vi "IMAQController.ReadConfigFile.vi"(0 "object ref in":refnum<vi>, 5 "error in":errorcluster) -> (14 "object ref out":refnum<vi>, 16 "Camera-System Configuration":T1(array[cluster]), 19 "error out":errorcluster)   [LabVIEW 2014, in "IMAQController.lvlib"]
uses:
  IMAQController.lvlib
  CSCore/BaseProcess/BaseProcess.lvlib
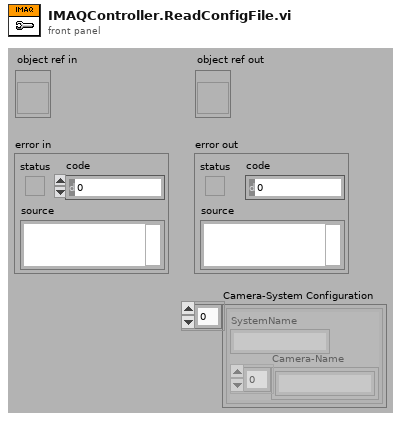
[diagram p1: front panel]
types:
  T1 = cluster{"SystemName":string, "Camera-Name":string[]}[]
  T2 = cluster{"SystemName":string, "Camera-Name":string[]}
  T3 = typedef "BaseProcess.lvlib/BaseProcess.i attribute.ctl" = cluster{"EventStatus":string, "EventError":i32, "PresetEvtWatchD":i32, "PresetPdcWatchD":i32, "EventTimeout":i32, "PeriodicInterval":i32, "Interface":string[], "Address":string[], "Special":string[], "PeriodicError":i32, "PeriodicStatus":string, "SuperProc":string, "Descriptors":T4[], "CaseRef":refnum<vi>, "PdcRef":refnum<vi>, "Thread Ref":refnum<vi>, "eventErrorID":i32, "eventStatusID":i32, "periodicErrorID":i32, "periodicStatusID":i32, "pdcCtrID":i32}
  T4 = typedef "BaseProcess.lvlib/BaseProcess.descriptor definition.ctl" = cluster{"selector":string, "descriptor":T5}
  T5 = typedef "BaseProcess.lvlib/BaseProcess.descriptor string definition.ctl" = string
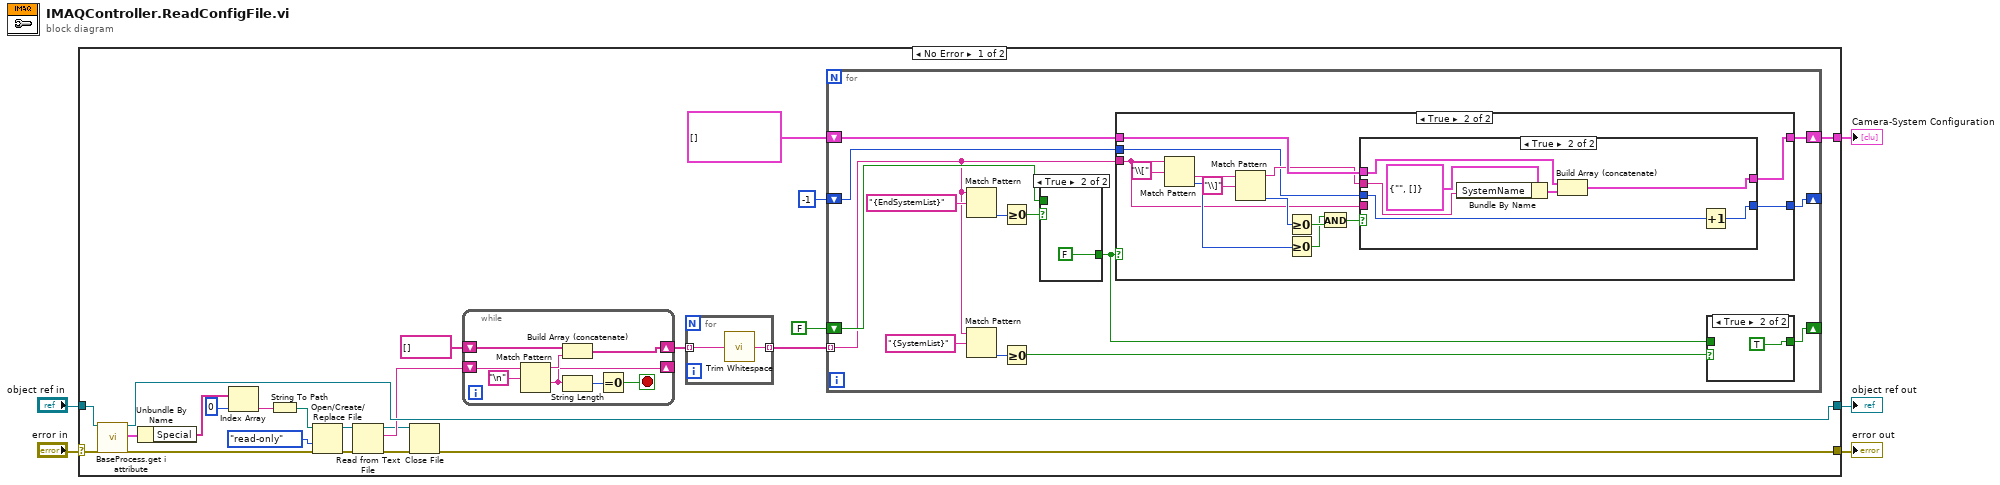
[diagram p0: block diagram]
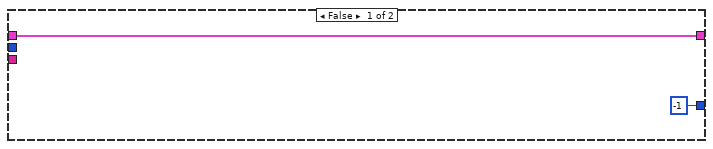
[diagram p2: hidden frame]
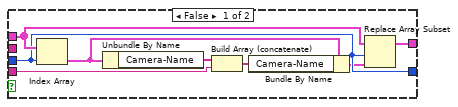
[diagram p3: hidden frame]
diagram:
  n1 = case shown="No Error" "error in" {
    selector: "error in" -> [w27 w89]
    tunnel: "object ref in" -> [w28 w88]
    tunnel: [w11 w89] -> w3
    tunnel: [w22 w88] -> w2
    tunnel: [w6 _] -> w1
    frame No Error {
      n2 = call "BaseProcess.get i attribute.vi"("i ref in"=w28, "error in (no error)"=w27) -> ("i ref out"=w22:refnum<vi>, "i attribute"=w26:T3, "error out"=w21:errorcluster)  [unwired: 15 in]
      n3 = Unbundle By Name(w26) -> ("Special"=w25:string[])
      n4 = Index Array(array=w25, index=0) -> (element=w23:string)
      n5 = String To Path(string=w23) -> (path=w20:path)
      n6 = Open/Create/Replace File(file path (use dialog)=w20, error in=w21, access (0:read/write)=enum16{"read/write", "read-only", "write-only"}."read-only") -> (refnum out=w17:refnum<file>, error out=w18:errorcluster)  [unwired: 3 in, 1 out]
      n7 = Read from Text File(file (use dialog)=w17, error in=w18) -> (refnum out=w13:refnum<file>, text=w15:string, error out=w12:errorcluster)  [unwired: 2 in, 1 out]
      n8 = Close File(refnum=w13, error in=w12) -> (error out=w11:errorcluster)  [unwired: 1 out]
      n9 = while {
        shift-right: [w82] -> _
        shift-left: w15 -> [w87]
        shift-right: [w84] -> w14
        shift-left: string[] [] -> [w85]
        stop <- w80 stop-if-true
        n10 = Match Pattern(string=w87, regular expression="\n") -> (before substring=w83:string, after substring=w82:string)  [unwired: 1 in, 2 out]
        n11 = Build Array (concatenate)(w85, w83) -> (w84:string[])
        n12 = String Length(string=w82) -> (length=w81:i32)
        n13 = Equal To 0?(x=w81) -> (x = 0?=w80:bool)
      }
      n14 = for {
        tunnel: w14 -> [w79] mode=indexing
        tunnel: [w78] -> w10 mode=indexing
        n15 = call <vilib>:"Trim Whitespace.vi"("string"=w79) -> ("trimmed string"=w78:string)  [unwired: 1 in]
      }
      n16 = for {
        tunnel: w10 -> [w33] mode=indexing
        shift-right: [w39] -> _
        shift-left: FALSE -> [w35]
        shift-right: [w31] -> w6
        shift-left: T1 [] ("Camera-System Configuration") -> [w32]
        shift-right: [w29] -> _
        shift-left: -1 -> [w30]
        n17 = Match Pattern(string=w33, regular expression="{EndSystemList}") -> (offset past match=w36:i32)  [unwired: 1 in, 3 out]
        n18 = Match Pattern(string=w33, regular expression="{SystemList}") -> (offset past match=w41:i32)  [unwired: 1 in, 3 out]
        n19 = Greater Or Equal To 0?(x=w36) -> (x >= 0?=w38:bool)
        n20 = Greater Or Equal To 0?(x=w41) -> (x >= 0?=w40:bool)
        n21 = case shown="True" w38 {
          tunnel: w35 -> [w74 _]
          tunnel: [w74 FALSE] -> w34
          frame False {
          }
          frame True {
          }
        }
        n22 = case shown="True" w34 {
          tunnel: w33 -> [_ w45]
          tunnel: w32 -> [w44 w50]
          tunnel: [w44 w49] -> w31
          tunnel: w30 -> [_ w47]
          tunnel: [-1 w46] -> w29
          frame False {
          }
          frame True {
            n23 = Match Pattern(string=w45, regular expression="\\[") -> (after substring=w58:string, offset past match=w55:i32)  [unwired: 1 in, 2 out]
            n24 = Match Pattern(string=w58, regular expression="\\]") -> (before substring=w48:string, offset past match=w54:i32)  [unwired: 1 in, 2 out]
            n25 = Greater Or Equal To 0?(x=w54) -> (x >= 0?=w53:bool)
            n26 = Greater Or Equal To 0?(x=w55) -> (x >= 0?=w52:bool)
            n27 = And(x=w52, y=w53) -> (x .and. y?=w51:bool)
            n28 = case shown="True" w51 {
              tunnel: w50 -> [w65 w73]
              tunnel: [w66 w72] -> w49
              tunnel: w48 -> [_ w69]
              tunnel: w47 -> [w64 w68]
              tunnel: [w64 w67] -> w46
              tunnel: w45 -> [w60 _]
              frame False {
                n29 = Index Array(array=w65, index=w64) -> (element=w62:T2)
                n30 = Unbundle By Name(w62) -> ("Camera-Name"=w61:string[])
                n31 = Build Array (concatenate)(w61, w60) -> (w59:string[])
                n32 = Bundle By Name(cluster=w62, "Camera-Name"=w59) -> (w63:T2)
                n33 = Replace Array Subset(array=w65, new element=w63, index=w64) -> (w66:T1)
              }
              frame True {
                n34 = Bundle By Name(cluster=T2 {"SystemName"="", "Camera-Name"=[]}, "SystemName"=w69) -> (w71:T2)
                n35 = Build Array (concatenate)(w73, w71) -> (w72:T1)
                n36 = Increment(x=w68) -> (x+1=w67:i32)
              }
            }
          }
        }
        n37 = case shown="True" w40 {
          tunnel: w34 -> [w76 _]
          tunnel: [w76 TRUE] -> w39
          frame False {
          }
          frame True {
          }
        }
      }
    }
    frame Error {
    }
  }
  "error out" <- w3
  "object ref out" <- w2
  "Camera-System Configuration" <- w1
